vi "Kinect Save Baseline Image.vi"(8 "error in (no error)":errorcluster, 10 "Baseline Image Path":path, 11 "Baseline Image":T1) -> (0 "error out":errorcluster, 3 "Baseline Image Out":T1)   [LabVIEW 2011]
uses:
  <vilib>/vision/Image Controls.llb/IMAQ Image.ctl
  <vilib>/vision/NI_Vision_Development_Module.lvlib
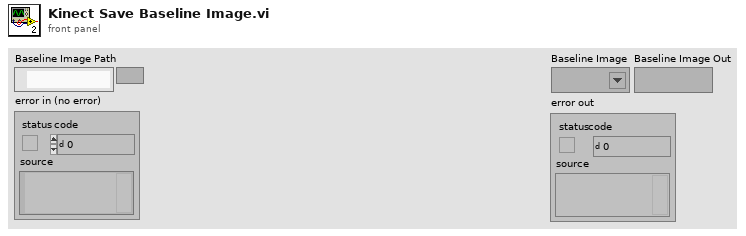
[diagram p1: front panel]
types:
  T1 = typedef "IMAQ Image.ctl" = refnum<image>
  T2 = typedef "Image Type" = u32
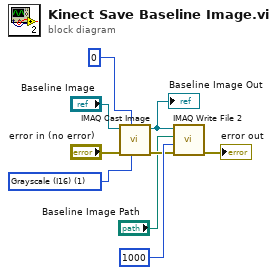
[diagram p0: block diagram]
diagram:
  w9 = T2 1 items=["Grayscale (U8)", "Grayscale (I16)", "Grayscale (SGL)", "Complex (CSG)", "RGB (U32)", "HSL (U32)", "RGB (U64)", "Grayscale (U16)"] ("Image Type")
  n1 = call "IMAQ Cast Image"("Image Type"=w9, "# Shifts"=0, "error in (no error)"="error in (no error)", "Image Src"="Baseline Image") -> ("error out"=w6:errorcluster, "Image Dst Out"=w3:T1)  [unwired: 6 in]
  "Baseline Image Out" <- w3
  n2 = call-poly "IMAQ Write File 2"("error in (no error)"=w6, "Image Quality"=u32 1000, "File Path"="Baseline Image Path", "Image"=w3) -> ("error out"=→"error out":errorcluster)  [unwired: 6 in, 1 out]
